vi "templates save template.vi"(6 "sxUsername":string, 7 "Post Parameters In":T1, 8 "error in (no error)":errorcluster, 10 "sxTemplateId":string, 11 "Connection Refnum":T3) -> (0 "error out":errorcluster, 1 "template parameters":T1, 2 "New Template Record":T2, 3 "Connection Refnum":T3, 5 "Post Parameters Out":T1)   [LabVIEW 2011]
uses:
  Addons/internet/utils/keyedarr.llb/Keyed Array.ctl
  SI.LIB/ODBC/SQL Controls/Connection Refnum.ctl
  server/database/Templates/Template Record.ctl
  Addons/internet/utils/strutil.llb/Case Matching.ctl
panel:
  out "KEYS and VALUES":T1
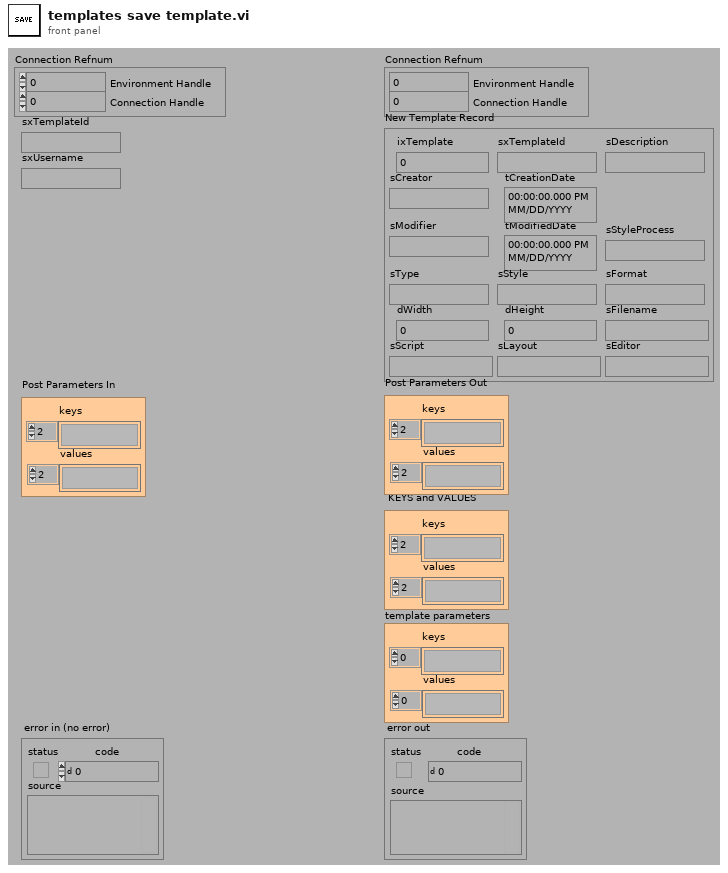
[diagram p1: front panel]
types:
  T1 = typedef "Keyed Array.ctl" = cluster{"keys":string[], "values":string[]}
  T2 = typedef "Template Record.ctl" = cluster{"ixTemplate":i32, "sxTemplateId":string, "sDescription":string, "sCreator":string, "tCreationDate":timestamp, "sModifier":string, "tModifiedDate":timestamp, "sType":string, "sStyle":string, "sFormat":string, "dWidth":dbl, "dHeight":dbl, "sFilename":string, "sScript":string, "sLayout":string, "sEditor":string, "sStyleProcess":string}
  T3 = typedef "Connection Refnum.ctl" = cluster{"Environment Handle":i32, "Connection Handle":i32}
  T4 = typedef "Case Matching.ctl" = enum16{"a != A", "a == A", "system"}
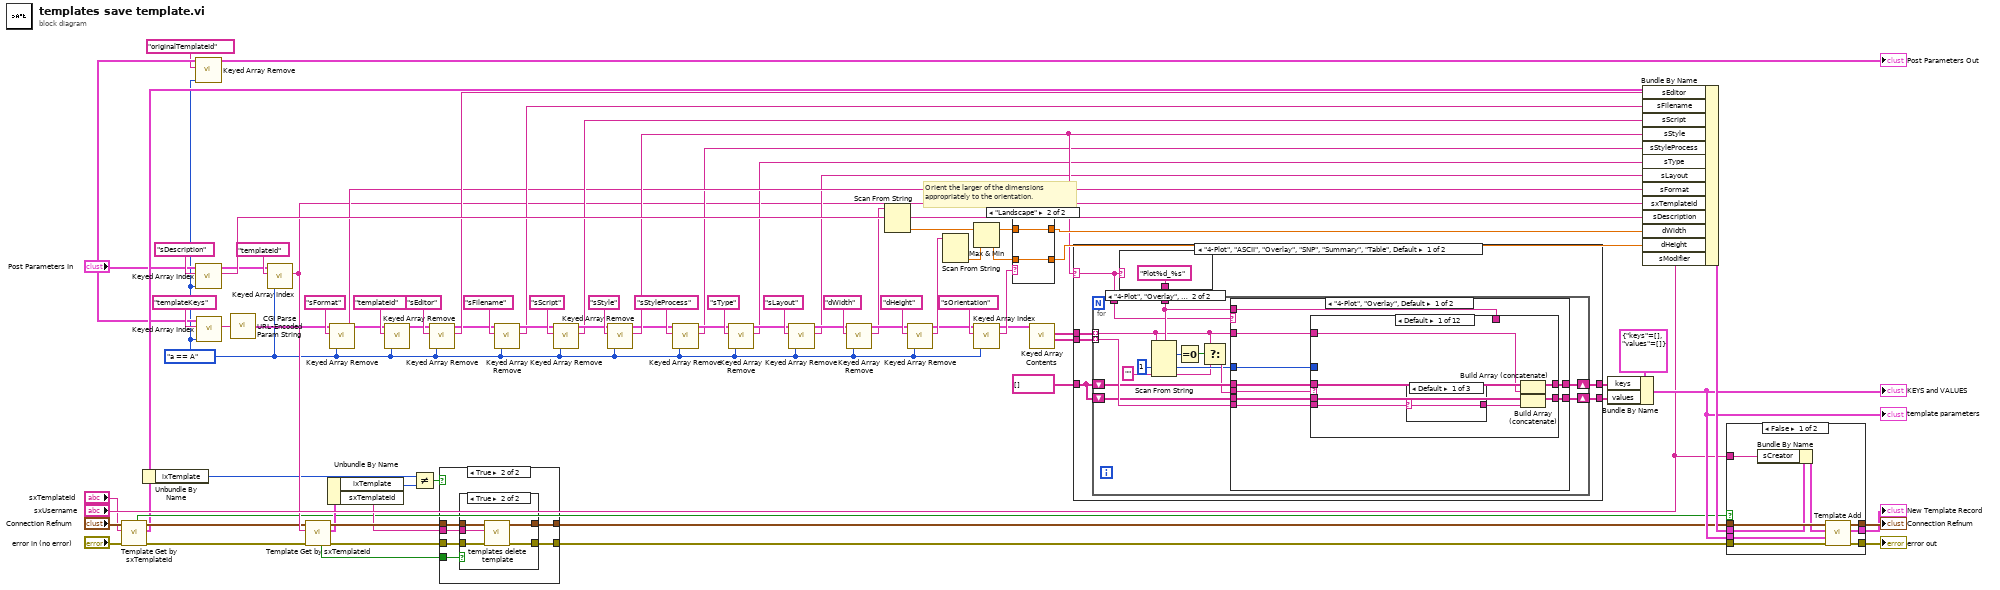
[diagram p0: block diagram]
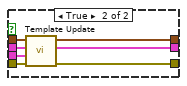
[diagram p4: hidden frame]
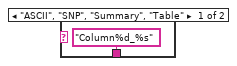
[diagram p5: hidden frame]
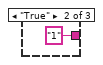
[diagram p6: hidden frame]
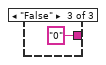
[diagram p7: hidden frame]
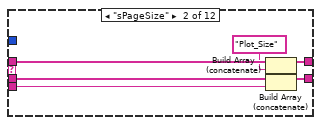
[diagram p8: hidden frame]
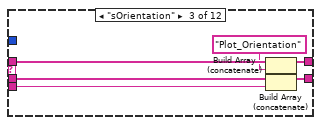
[diagram p9: hidden frame]
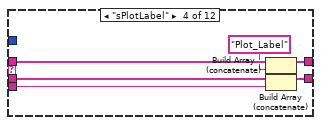
[diagram p10: hidden frame]
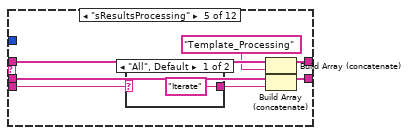
[diagram p11: hidden frame]
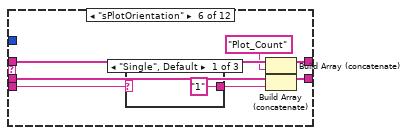
[diagram p13: hidden frame]
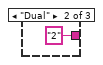
[diagram p14: hidden frame]
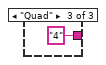
[diagram p15: hidden frame]
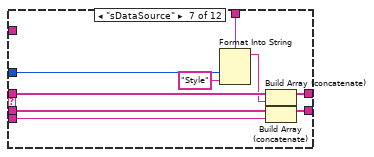
[diagram p16: hidden frame]
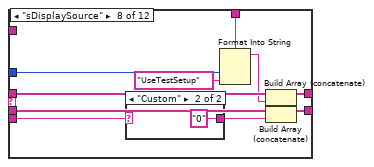
[diagram p17: hidden frame]
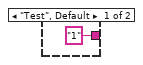
[diagram p18: hidden frame]
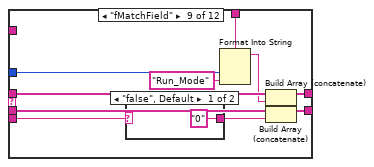
[diagram p19: hidden frame]
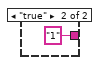
[diagram p20: hidden frame]
diagram:
  w2 = Case_Matching."a == A" ("case matching (sensitive)")
  # "Orient the larger of the dimensions\nappropriately to the orientation."
  n1 = call "Template Get by sxTemplateId.vi"("error in (no error)"="error in (no error)", "sxTemplateId (\"\")"="sxTemplateId", "Connection Refnum"="Connection Refnum") -> ("error out"=w11:errorcluster, "Template Record"=w6:T2, "Connection Refnum"=w12:T3, "Data Present"=w9:bool)  [unwired: 5 out]
  n2 = Unbundle By Name(w6) -> ("ixTemplate"=w5:i32)
  n3 = call "Keyed Array Remove.vi"("case matching (sensitive)"=w2, "key"="originalTemplateId", "array in"="Post Parameters In") -> ("array out"=→"Post Parameters Out":T1)  [unwired: 4 out]
  n4 = call "Keyed Array Index.vi"("case matching (sensitive)"=w2, "key"="sDescription", "array in"="Post Parameters In") -> ("value"=w77:string, "duplicate array"=w29:T1)  [unwired: 1 in, 2 out]
  n5 = call "Keyed Array Index.vi"("case matching (sensitive)"=w2, "key"="templateKeys", "array in"="Post Parameters In") -> ("value"=w28:string)  [unwired: 1 in, 3 out]
  n6 = call "CGI Parse URL-Encoded Param String.vi"("url-encoded param string"=w28) -> ("params"=w39:T1)
  n7 = call "Keyed Array Index.vi"("case matching (sensitive)"=w2, "key"="templateId", "array in"=w29) -> ("value"=w22:string)  [unwired: 1 in, 3 out]
  n8 = call "Template Get by sxTemplateId.vi"("error in (no error)"=w11, "sxTemplateId (\"\")"=w22, "Connection Refnum"=w12) -> ("error out"=w21:errorcluster, "Template Record"=w17:T2, "Connection Refnum"=w20:T3, "Data Present"=w15:bool)  [unwired: 5 out]
  n9 = Unbundle By Name(w17) -> ("ixTemplate"=w8:i32, "sxTemplateId"=w16:string)
  n10 = call "Keyed Array Remove.vi"("case matching (sensitive)"=w2, "key"="sFormat", "array in"=w39) -> ("value"=w37:string, "array out"=w38:T1)  [unwired: 3 out]
  n11 = call "Keyed Array Remove.vi"("case matching (sensitive)"=w2, "key"="templateId", "array in"=w38) -> ("array out"=w48:T1)  [unwired: 4 out]
  n12 = Not Equal?(x=w5, y=w8) -> (x != y?=w7:bool)
  n13 = call "Keyed Array Remove.vi"("case matching (sensitive)"=w2, "key"="sEditor", "array in"=w48) -> ("value"=w50:string, "array out"=w45:T1)  [unwired: 3 out]
  n14 = case shown="True" w7 {
    tunnel: [w84 w90] -> w19
    tunnel: [w83 w89] -> w18
    tunnel: w16 -> [_ w88]
    tunnel: w21 -> [w83 w87]
    tunnel: w20 -> [w84 w86]
    tunnel: w15 -> [_ w85]
    frame False {
    }
    frame True {
      n15 = case shown="True" w85 {
        tunnel: w86 -> [w92 w97]
        tunnel: [w92 w96] -> w90
        tunnel: w87 -> [w91 w95]
        tunnel: w88 -> [_ w94]
        tunnel: [w91 w93] -> w89
        frame False {
        }
        frame True {
          n16 = call "templates delete template.vi"("error in (no error)"=w95, "sxTemplateId (\"\")"=w94, "Connection Refnum In\n(0,0: Open New)"=w97) -> ("error out"=w93:errorcluster, "Connection Refnum In\n(0,0: Open New)"=w96:T3)  [unwired: 7 out]
        }
      }
    }
  }
  n17 = call "Keyed Array Remove.vi"("case matching (sensitive)"=w2, "key"="sFilename", "array in"=w45) -> ("value"=w41:string, "array out"=w44:T1)  [unwired: 3 out]
  n18 = call "Keyed Array Remove.vi"("case matching (sensitive)"=w2, "key"="sScript", "array in"=w44) -> ("value"=w42:string, "array out"=w43:T1)  [unwired: 3 out]
  n19 = call "Keyed Array Remove.vi"("case matching (sensitive)"=w2, "key"="sStyle", "array in"=w43) -> ("value"=w52:string, "array out"=w26:T1)  [unwired: 3 out]
  n20 = call "Keyed Array Remove.vi"("case matching (sensitive)"=w2, "key"="sStyleProcess", "array in"=w26) -> ("value"=w24:string, "array out"=w25:T1)  [unwired: 3 out]
  n21 = call "Keyed Array Remove.vi"("case matching (sensitive)"=w2, "key"="sType", "array in"=w25) -> ("value"=w32:string, "array out"=w34:T1)  [unwired: 3 out]
  n22 = call "Keyed Array Remove.vi"("case matching (sensitive)"=w2, "key"="sLayout", "array in"=w34) -> ("value"=w31:string, "array out"=w33:T1)  [unwired: 3 out]
  n23 = call "Keyed Array Remove.vi"("case matching (sensitive)"=w2, "key"="dWidth", "array in"=w33) -> ("value"=w73:string, "array out"=w74:T1)  [unwired: 3 out]
  n24 = Scan From String(input string=w73) -> (output 1=w58:dbl)  [unwired: 3 in, 4 out]
  n25 = call "Keyed Array Remove.vi"("case matching (sensitive)"=w2, "key"="dHeight", "array in"=w74) -> ("value"=w72:string, "array out"=w70:T1)  [unwired: 3 out]
  n26 = Scan From String(input string=w72) -> (output 1=w57:dbl)  [unwired: 3 in, 4 out]
  n27 = Max & Min(x=w58, y=w57) -> (max(x,y)=w55:dbl, min(x,y)=w56:dbl)
  n28 = call "Keyed Array Index.vi"("case matching (sensitive)"=w2, "key"="sOrientation", "array in"=w70) -> ("value"=w69:string, "duplicate array"=w66:T1)  [unwired: 1 in, 2 out]
  n29 = case shown="\"Landscape\"" w69 {
    tunnel: w56 -> [w99 w100]
    tunnel: w55 -> [w98 w101]
    tunnel: [w99 w101] -> w68
    tunnel: [w98 w100] -> w67
    frame "Portrait", Default {
    }
    frame "Landscape" {
    }
  }
  n30 = call "Keyed Array Contents.vi"("array in"=w66) -> ("values"=w64:string[], "keys"=w65:string[])  [unwired: 5 out]
  n31 = case shown="\"4-Plot\", \"ASCII\", \"Overlay\", \"SNP\", \"Summary\", \"Table\", Default" w52 {
    selector: w52 -> [w102 _]
    tunnel: w65 -> [w108 w376]
    tunnel: w64 -> [w107 w375]
    tunnel: string[] [] -> [w106 w374]
    tunnel: [w105 w373] -> w61
    tunnel: [w104 w372] -> w60
    frame "4-Plot", "ASCII", "Overlay", "SNP", "Summary", "Table", Default {
      n32 = case shown="\"4-Plot\", \"Overlay\", Default" w102 {
        tunnel: ["Column%d_%s" ("regular expression") "Plot%d_%s" ("regular expression")] -> w103
        frame "ASCII", "SNP", "Summary", "Table" {
        }
        frame "4-Plot", "Overlay", Default {
        }
      }
      n33 = for {
        tunnel: w108 -> [w112] mode=indexing
        tunnel: w107 -> [w125] mode=indexing
        shift-right: [w122] -> w105
        shift-left: w106 -> [w124]
        shift-right: [w121] -> w104
        shift-left: w106 -> [w123]
        tunnel: w103 -> [w117]
        tunnel: w102 -> [w111]
        n34 = Scan From String(format string=w117, input string=w112, default 1=1, default 2="" ("regular expression")) -> (offset past scan=w114:u32, output 1=w116:i32, output 2=w113:string)  [unwired: 2 in, 2 out]
        n35 = Equal To 0?(x=w114) -> (x = 0?=w120:bool)
        n36 = Select(t=w112, s=w120, f=w113) -> (s? t:f=w119:string)
        n37 = case shown="\"4-Plot\", \"Overlay\", Default" w111 {
          tunnel: w125 -> [w134 w253]
          tunnel: w124 -> [w133 w252]
          tunnel: w123 -> [w132 w251]
          tunnel: [w131 w250] -> w122
          tunnel: [w130 w249] -> w121
          tunnel: w119 -> [w129 w248]
          tunnel: w117 -> [w128 w247]
          tunnel: w116 -> [w127 w246]
          tunnel: w112 -> [w126 w245]
          frame "4-Plot", "Overlay", Default {
            n38 = case shown="Default" w129 {
              tunnel: w134 -> [w136 w145 w151 w157 w164 w178 w182 w195 w204 w221 w230 w237]
              tunnel: w133 -> [w141 w150 w156 w162 w169 w177 w190 w200 w212 w215 w224 w242]
              tunnel: w132 -> [w140 w149 w155 w161 w168 w176 w189 w199 w211 w216 w225 w241]
              tunnel: [w139 w148 w154 w160 w167 w173 w188 w198 w210 w223 w232 w240] -> w131
              tunnel: [w138 w147 w153 w159 w166 w172 w187 w197 w209 w222 w231 w239] -> w130
              tunnel: w126 -> [w135 _ _ _ _ _ _ _ _ _ _ _]
              tunnel: w128 -> [_ _ _ _ _ _ w183 w192 w205 w217 w226 w236]
              tunnel: w127 -> [_ _ _ _ _ _ w185 w191 w206 w218 w227 w235]
              frame Default {
                n39 = case shown="Default" w136 {
                  selector: w136 -> [w142 _ _]
                  tunnel: [w142 "1" ("section") "0" ("section")] -> w137
                  frame Default {
                  }
                  frame "True" {
                  }
                  frame "False" {
                  }
                }
                n40 = Build Array (concatenate)(w141, w135) -> (w139:string[])
                n41 = Build Array (concatenate)(w140, w137) -> (w138:string[])
              }
              frame "sPageSize" {
                n42 = Build Array (concatenate)(w150, "Plot_Size" ("section")) -> (w148:string[])
                n43 = Build Array (concatenate)(w149, w145) -> (w147:string[])
              }
              frame "sOrientation" {
                n44 = Build Array (concatenate)(w156, "Plot_Orientation" ("section")) -> (w154:string[])
                n45 = Build Array (concatenate)(w155, w151) -> (w153:string[])
              }
              frame "sPlotLabel" {
                n46 = Build Array (concatenate)(w162, "Plot_Label" ("section")) -> (w160:string[])
                n47 = Build Array (concatenate)(w161, w157) -> (w159:string[])
              }
              frame "sResultsProcessing" {
                n48 = case shown="\"All\", Default" w164 {
                  selector: w164 -> [_ w171]
                  tunnel: ["Iterate" ("section") w171] -> w163
                  frame "All", Default {
                  }
                  frame "Most Recent" {
                  }
                }
                n49 = Build Array (concatenate)(w169, "Template_Processing" ("section")) -> (w167:string[])
                n50 = Build Array (concatenate)(w168, w163) -> (w166:string[])
              }
              frame "sPlotOrientation" {
                n51 = case shown="\"Single\", Default" w178 {
                  tunnel: ["1" ("section") "2" ("section") "4" ("section")] -> w175
                  frame "Single", Default {
                  }
                  frame "Dual" {
                  }
                  frame "Quad" {
                  }
                }
                n52 = Build Array (concatenate)(w177, "Plot_Count" ("section")) -> (w173:string[])
                n53 = Build Array (concatenate)(w176, w175) -> (w172:string[])
              }
              frame "sDataSource" {
                n54 = Format Into String(format string=w183, w185, "Style" ("section")) -> (resulting string=w184:string)  [unwired: 2 in, 1 out]
                n55 = Build Array (concatenate)(w190, w184) -> (w188:string[])
                n56 = Build Array (concatenate)(w189, w182) -> (w187:string[])
              }
              frame "sDisplaySource" {
                n57 = case shown="\"Custom\"" w195 {
                  tunnel: ["1" ("section") "0" ("section")] -> w196
                  frame "Test", Default {
                  }
                  frame "Custom" {
                  }
                }
                n58 = Format Into String(format string=w192, w191, "UseTestSetup" ("section")) -> (resulting string=w193:string)  [unwired: 2 in, 1 out]
                n59 = Build Array (concatenate)(w200, w193) -> (w198:string[])
                n60 = Build Array (concatenate)(w199, w196) -> (w197:string[])
              }
              frame "fMatchField" {
                n61 = case shown="\"false\", Default" w204 {
                  tunnel: ["0" ("section") "1" ("section")] -> w203
                  frame "false", Default {
                  }
                  frame "true" {
                  }
                }
                n62 = Format Into String(format string=w205, w206, "Run_Mode" ("section")) -> (resulting string=w207:string)  [unwired: 2 in, 1 out]
                n63 = Build Array (concatenate)(w212, w207) -> (w210:string[])
                n64 = Build Array (concatenate)(w211, w203) -> (w209:string[])
              }
              frame "sFieldName" {
                n65 = Format Into String(format string=w217, w218, "Run_Field" ("section")) -> (resulting string=w219:string)  [unwired: 2 in, 1 out]
                n66 = Build Array (concatenate)(w215, w219) -> (w223:string[])
                n67 = Build Array (concatenate)(w216, w221) -> (w222:string[])
              }
              frame "sFieldValue" {
                n68 = Format Into String(format string=w226, w227, "Run_Field_Value" ("section")) -> (resulting string=w228:string)  [unwired: 2 in, 1 out]
                n69 = Build Array (concatenate)(w224, w228) -> (w232:string[])
                n70 = Build Array (concatenate)(w225, w230) -> (w231:string[])
              }
              frame "sLineType" {
                n71 = case shown="\"Symbols\"" w237 {
                  tunnel: ["0" ("section") "1" ("section")] -> w238
                  frame "Colors", Default {
                  }
                  frame "Symbols" {
                  }
                }
                n72 = Format Into String(format string=w236, w235, "LineType" ("section")) -> (resulting string=w233:string)  [unwired: 2 in, 1 out]
                n73 = Build Array (concatenate)(w242, w233) -> (w240:string[])
                n74 = Build Array (concatenate)(w241, w238) -> (w239:string[])
              }
            }
          }
          frame "ASCII", "SNP", "Summary", "Table" {
            n75 = case shown="Default" w248 {
              tunnel: w253 -> [w255 w264 w270 w277 w283 w294 w303 w321 w336 w343 w363]
              tunnel: w252 -> [w260 w269 w275 w281 w291 w302 w311 w320 w330 w347 w369]
              tunnel: w251 -> [w259 w268 w274 w280 w290 w301 w310 w319 w335 w355 w366]
              tunnel: [w258 w267 w273 w279 w289 w300 w309 w320 w330 w347 w368] -> w250
              tunnel: [w257 w266 w272 w278 w288 w299 w308 w318 w334 w354 w367] -> w249
              tunnel: w245 -> [w254 _ _ _ _ _ _ _ _ _ _]
              tunnel: w247 -> [_ _ _ _ w284 w295 w304 w315 w329 w344 w365]
              tunnel: w246 -> [_ _ _ _ w285 w296 w305 w314 w328 w345 w364]
              frame Default {
                n76 = case shown="Default" w255 {
                  selector: w255 -> [w261 _ _]
                  tunnel: [w261 "1" ("section") "0" ("section")] -> w256
                  frame Default {
                  }
                  frame "True" {
                  }
                  frame "False" {
                  }
                }
                n77 = Build Array (concatenate)(w260, w254) -> (w258:string[])
                n78 = Build Array (concatenate)(w259, w256) -> (w257:string[])
              }
              frame "sPageSize" {
                n79 = Build Array (concatenate)(w269, "Plot_Size" ("section")) -> (w267:string[])
                n80 = Build Array (concatenate)(w268, w264) -> (w266:string[])
              }
              frame "sOrientation" {
                n81 = Build Array (concatenate)(w275, "Plot_Orientation" ("section")) -> (w273:string[])
                n82 = Build Array (concatenate)(w274, w270) -> (w272:string[])
              }
              frame "sTableLabel" {
                n83 = Build Array (concatenate)(w281, "Table_Label" ("section")) -> (w279:string[])
                n84 = Build Array (concatenate)(w280, w277) -> (w278:string[])
              }
              frame "sRunSelection" {
                n85 = case shown="\"Match Field\"" w283 {
                  selector: w283 -> [w292 _ _]
                  tunnel: [w292 "Test_Run=" ("section") _] -> w282
                  frame "Most Recent", Default {
                  }
                  frame "Test Run" {
                  }
                  frame "Match Field" {
                  }
                }
                n86 = Format Into String(format string=w284, w285, "Run" ("section")) -> (resulting string=w286:string)  [unwired: 2 in, 1 out]
                n87 = Build Array (concatenate)(w291, w286) -> (w289:string[])
                n88 = Build Array (concatenate)(w290, w282) -> (w288:string[])
              }
              frame "sType" {
                n89 = Format Into String(format string=w295, w296, "Type" ("section")) -> (resulting string=w297:string)  [unwired: 2 in, 1 out]
                n90 = Build Array (concatenate)(w302, w297) -> (w300:string[])
                n91 = Build Array (concatenate)(w301, w294) -> (w299:string[])
              }
              frame "sLabel" {
                n92 = Format Into String(format string=w304, w305, "Label" ("section")) -> (resulting string=w306:string)  [unwired: 2 in, 1 out]
                n93 = Build Array (concatenate)(w311, w306) -> (w309:string[])
                n94 = Build Array (concatenate)(w310, w303) -> (w308:string[])
              }
              frame "dRunNumber" {
                n95 = Format Into String(format string=w315, w314, "Run" ("section")) -> (resulting string=w312:string)  [unwired: 2 in, 1 out]
                n96 = Search 1D Array(1D array=w320, element=w312) -> (index of element=w316:i32)  [unwired: 1 out]
                n97 = Index Array(array=w319, index=w316) -> (element=w322:string)
                n98 = case shown="Default" w322 {
                  selector: w322 -> [w323 w326]
                  tunnel: w321 -> [_ w325]
                  tunnel: [w323 w324] -> w317
                  frame Default {
                  }
                  frame "Test_Run=" {
                    n99 = Concatenate Strings(w326, w325) -> (w324:string)
                  }
                }
                n100 = Replace Array Subset(array=w319, new element=w317, index=w316) -> (w318:string[])
              }
              frame "sField" {
                n101 = Format Into String(format string=w329, w328, "Run" ("section")) -> (resulting string=w331:string)  [unwired: 2 in, 1 out]
                n102 = Search 1D Array(1D array=w330, element=w331) -> (index of element=w327:i32)  [unwired: 1 out]
                n103 = Index Array(array=w335, index=w327) -> (element=w337:string)
                n104 = case shown="\"\"" w337 {
                  selector: w337 -> [w338 _]
                  tunnel: w336 -> [_ w340]
                  tunnel: [w338 w341] -> w333
                  frame Default {
                  }
                  frame "" {
                    n105 = Concatenate Strings(w340, "=" ("section")) -> (w341:string)
                  }
                }
                n106 = Replace Array Subset(array=w335, new element=w333, index=w327) -> (w334:string[])
              }
              frame "sFieldValue" {
                n107 = case shown="Default" w343 {
                  selector: w343 -> [w356 _ _]
                  tunnel: [w356 "1" ("section") "0" ("section")] -> w342
                  frame Default {
                  }
                  frame "True" {
                  }
                  frame "False" {
                  }
                }
                n108 = Format Into String(format string=w344, w345, "Run" ("section")) -> (resulting string=w348:string)  [unwired: 2 in, 1 out]
                n109 = Search 1D Array(1D array=w347, element=w348) -> (index of element=w346:i32)  [unwired: 1 out]
                n110 = Index Array(array=w355, index=w346) -> (element=w350:string)
                n111 = Match Pattern(string=w350, regular expression="=") -> (before substring=w351:string)  [unwired: 4 out]
                n112 = case shown="Default" w351 {
                  tunnel: w342 -> [_ w360]
                  tunnel: [w359 w362] -> w353
                  tunnel: w350 -> [w359 w361]
                  frame "Most Recent", "Test_Run" {
                  }
                  frame Default {
                    n113 = Concatenate Strings(w361, w360) -> (w362:string)
                  }
                }
                n114 = Replace Array Subset(array=w355, new element=w353, index=w346) -> (w354:string[])
              }
              frame "sParameters" {
                n115 = Format Into String(format string=w365, w364, "Parameters" ("section")) -> (resulting string=w370:string)  [unwired: 2 in, 1 out]
                n116 = Build Array (concatenate)(w369, w370) -> (w368:string[])
                n117 = Build Array (concatenate)(w366, w363) -> (w367:string[])
              }
            }
          }
        }
      }
    }
    frame "Analysis" {
      n118 = for {
        tunnel: w376 -> [w377] mode=indexing
        tunnel: w375 -> [w382] mode=indexing
        shift-right: [w379] -> w373
        shift-left: w374 -> [w381]
        shift-right: [w378] -> w372
        shift-left: w374 -> [w380]
        n119 = case shown="\"Autoscale\", \"sOrientation\", \"sPageSize\"" w377 {
          selector: w377 -> [w383 _ _]
          tunnel: w382 -> [w384 w398 _]
          tunnel: w381 -> [w389 w396 w416]
          tunnel: w380 -> [w388 w397 w415]
          tunnel: [w387 w394 w416] -> w379
          tunnel: [w386 w393 w415] -> w378
          frame Default {
            n120 = case shown="Default" w384 {
              selector: w384 -> [w390 _ _]
              tunnel: [w390 "1" ("section") "0" ("section")] -> w385
              frame Default {
              }
              frame "True" {
              }
              frame "False" {
              }
            }
            n121 = Build Array (concatenate)(w389, w383) -> (w387:string[])
            n122 = Build Array (concatenate)(w388, w385) -> (w386:string[])
          }
          frame "Parameter" {
            n123 = Search 1D Array(1D array=w396, element="Test_Type" ("section")) -> (index of element=w395:i32)  [unwired: 1 out]
            n124 = Index Array(array=w397, index=w395) -> (element=w399:string)
            n125 = case shown="\"Prompted Inputs\"" w399 {
              selector: w399 -> [w404 _]
              tunnel: w398 -> [w403 w410]
              tunnel: w397 -> [w408 w411]
              tunnel: w396 -> [w406 w414]
              tunnel: w395 -> [w407 _]
              tunnel: [w406 w413] -> w394
              tunnel: [w405 w412] -> w393
              frame "Prompted Inputs" {
                n126 = Concatenate Strings(w404, " " ("string"), w403) -> (w401:string)
                n127 = Replace Array Subset(array=w408, new element=w401, index=w407) -> (w405:string[])
              }
              frame Default {
                n128 = Build Array (concatenate)(w414, "Parameter" ("section")) -> (w413:string[])
                n129 = Build Array (concatenate)(w411, w410) -> (w412:string[])
              }
            }
          }
          frame "Autoscale", "sOrientation", "sPageSize" {
          }
        }
      }
    }
  }
  n130 = Bundle By Name(cluster=T1 {"keys"=[], "values"=[]} ("POST Parameters"), "keys"=w61, "values"=w60) -> (w59:T1)
  "KEYS and VALUES" <- w59
  "template parameters" <- w59
  n131 = Bundle By Name(cluster=w6, "sEditor"=w50, "sFilename"=w41, "sScript"=w42, "sStyle"=w52, "sStyleProcess"=w24, "sType"=w32, "sLayout"=w31, "sFormat"=w37, "sxTemplateId"=w22, "sDescription"=w77, "dWidth"=w68, "dHeight"=w67, "sModifier"="sxUsername") -> (w82:T2)
  n132 = case shown="False" w9 {
    tunnel: w18 -> [w424 w432]
    tunnel: w19 -> [w425 w431]
    tunnel: w82 -> [w419 w430]
    tunnel: [w423 w429] -> w81
    tunnel: [w422 w428] -> w80
    tunnel: w59 -> [w420 w427]
    tunnel: [w421 w426] -> w54
    tunnel: "sxUsername" -> [w417 _]
    frame False {
      n133 = Bundle By Name(cluster=w419, "sCreator"=w417) -> (w418:T2)
      n134 = call "Template Add.vi"("error in (no error)"=w424, "Parameters (empty)"=w420, "Template Record"=w418, "Connection Refnum"=w425) -> ("error out"=w423:errorcluster, "New Template Record"=w421:T2, "Connection Refnum"=w422:T3)  [unwired: 5 out]
    }
    frame True {
      n135 = call "Template Update.vi"("error in (no error)"=w432, "Parameters (empty)"=w427, "Template Record"=w430, "Connection Refnum"=w431) -> ("error out"=w429:errorcluster, "New Template Record"=w426:T2, "Connection Refnum"=w428:T3)  [unwired: 5 out]
    }
  }
  "error out" <- w81
  "Connection Refnum" <- w80
  "New Template Record" <- w54
